vi "Write Setpoint.vi"(8 "error in (no error)":errorcluster, 10 "ILC in":refnum<class "ILC.lvclass">, 11 "Actuator Cylinder in":refnum<class "Actuator Cylinder.lvclass">) -> (0 "error out":errorcluster, 2 "ILC out":refnum<class "ILC.lvclass">, 3 "Actuator Cylinder out":refnum<class "Actuator Cylinder.lvclass">)   [LabVIEW 2015, in "Actuator Cylinder.lvclass"]
uses:
  Actuator Cylinder.lvclass
  <userlib>/Common/ILC/ILC/ILC.lvclass
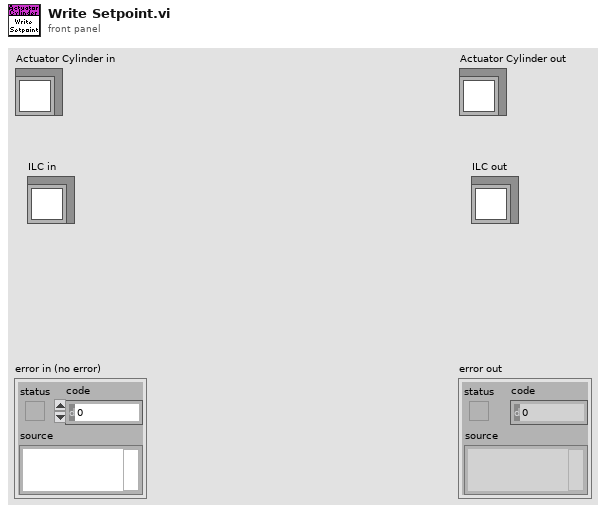
[diagram p1: front panel]
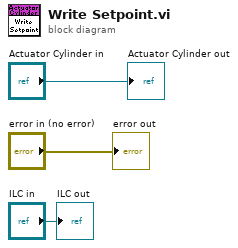
[diagram p0: block diagram]
diagram:
  "error out" <- "error in (no error)"
  "Actuator Cylinder out" <- "Actuator Cylinder in"
  "ILC out" <- "ILC in"
